vi "Tello Test.vi"(11 "Error in":errorcluster caption="Error in (no error)") -> (15 "Error out":errorcluster)   [LabVIEW 2020]
doc: "<Developer>\nGPower\n28/5 2020"
panel:
  out "data out 2":string
  out "data out":string
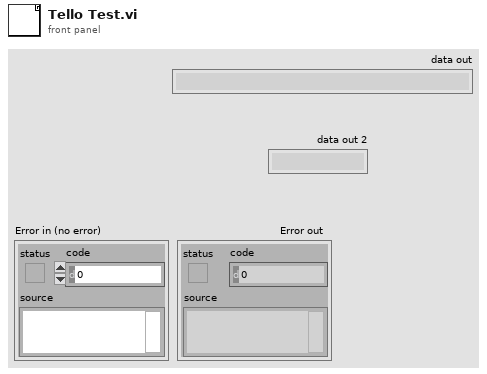
[diagram p1: front panel]
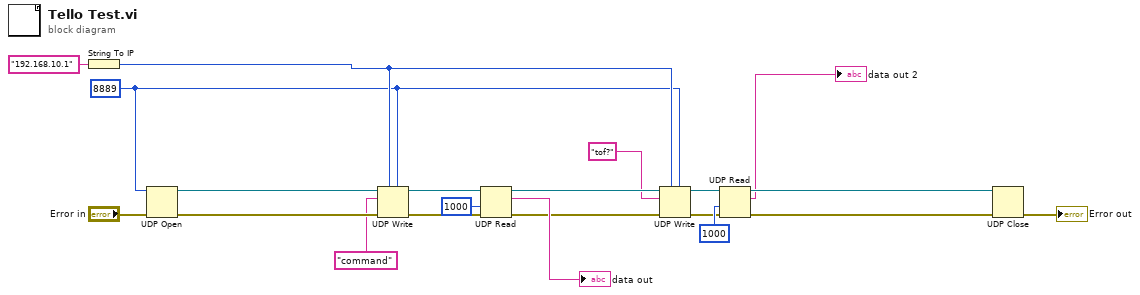
[diagram p0: block diagram]
diagram:
  w3 = u16 8889 ("port")
  n1 = String To IP(1:"192.168.10.1" ("name")) -> (0:w4:u32)
  n2 = UDP Open(8:"Error in", 11:w3) -> (port=w19:refnum<k16>, 0:w17:errorcluster)  [unwired: 3 in, 1 out]
  n3 = UDP Write(address=w4, port or service name=w3, connection ID=w19, data in="command", 8:w17) -> (error out=w16:errorcluster, 3:w18:refnum<k16>)  [unwired: 1 in]
  n4 = UDP Read(connection ID=w18, timeout ms (25000)=1000, 8:w16) -> (data out=→"data out":string, error out=w8:errorcluster, 3:w7:refnum<k16>)  [unwired: 1 in, 2 out]
  n5 = UDP Write(address=w4, port or service name=w3, connection ID=w7, data in="tof?", 8:w8) -> (error out=w9:errorcluster, 3:w10:refnum<k16>)  [unwired: 1 in]
  n6 = UDP Read(connection ID=w10, timeout ms (25000)=1000, 8:w9) -> (data out=→"data out 2":string, error out=w5:errorcluster, 3:w6:refnum<k16>)  [unwired: 1 in, 2 out]
  n7 = UDP Close(connection ID=w6, 8:w5) -> (error out=→"Error out":errorcluster)  [unwired: 1 out]
